vi "Migrate all Measurement Dependencies.vi"(0 "project path":path, 1 "measurement paths":path[](array[path]), 2 "init":T1[](array[typedef]), 5 "plug-in names":string[](array[string]), 7 "measurement dependencies":path[][](array[path]), 9 "outside items":string[](array[string]), 11 "error in":errorcluster, 12 "shared dependent vis":path[](array[path])) -> (6 "destination directory":path[](array[path]), 15 "error out":errorcluster)   [LabVIEW 2021, in "Multiple Converter.lvlib"]
uses:
  Multiple Converter.lvlib
  TypeDefs/Library Info.ctl
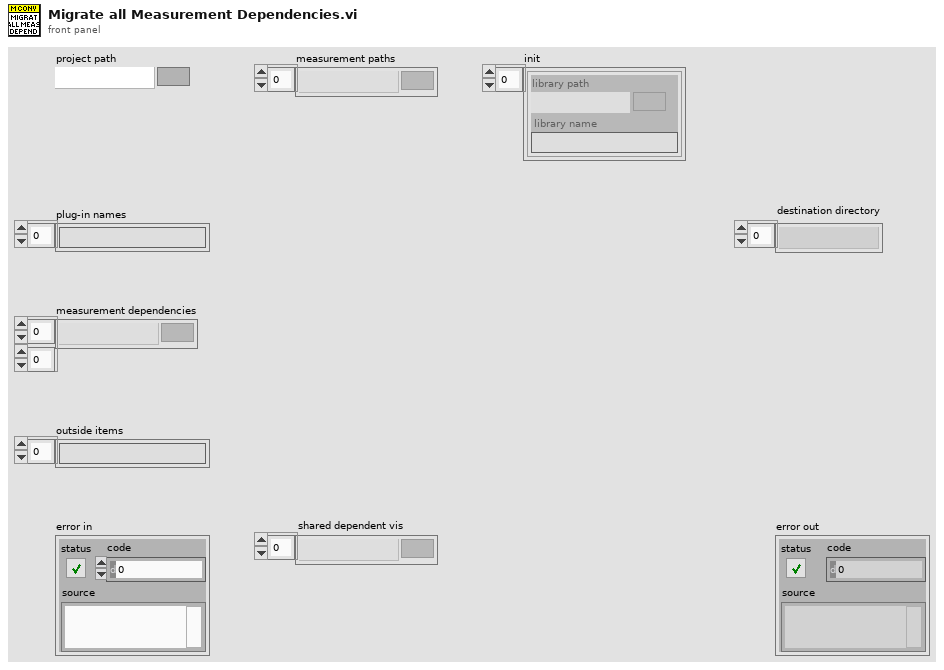
[diagram p1: front panel]
types:
  T1 = typedef "Multiple Converter.lvlib/Library Info.ctl" = cluster{"library path":path, "library name":string}
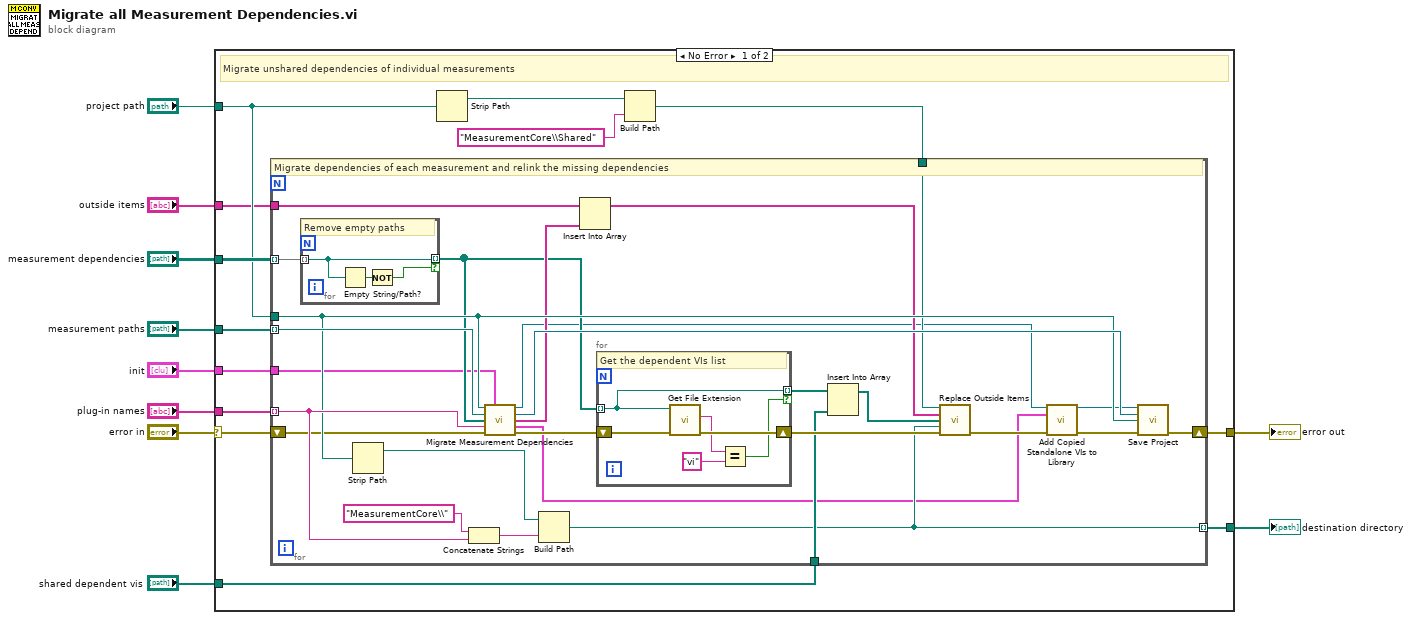
[diagram p0: block diagram]
diagram:
  n1 = case shown="No Error" "error in" {
    selector: "error in" -> [w22 w60]
    tunnel: "measurement dependencies" -> [w23 _]
    tunnel: "project path" -> [w18 _]
    tunnel: "outside items" -> [w17 _]
    tunnel: "measurement paths" -> [w16 _]
    tunnel: "plug-in names" -> [w15 _]
    tunnel: [w14 w60] -> w4
    tunnel: "shared dependent vis" -> [w13 _]
    tunnel: [w12 _] -> w2
    tunnel: "init" -> [w11 _]
    frame No Error {
      # "Migrate unshared dependencies of individual measurements"
      n2 = Strip Path(path=w18) -> (stripped path=w19:path)  [unwired: 1 out]
      n3 = Build Path(base path=w19, name or relative path="MeasurementCore\\Shared" ("string")) -> (appended path=w21:path)
      n4 = for {
        tunnel: w18 -> [w42]
        tunnel: w16 -> [w47] mode=indexing
        tunnel: w15 -> [w44] mode=indexing
        tunnel: w17 -> [w41]
        tunnel: w21 -> [w38]
        shift-right: [w48] -> w14
        shift-left: w22 -> [w37]
        tunnel: w23 -> [w36] mode=indexing
        tunnel: w13 -> [w31]
        tunnel: [w29] -> w12 mode=indexing
        tunnel: w11 -> [w28]
        # "Migrate dependencies of each measurement and relink the missing dependencies"
        n5 = for {
          tunnel: w36 -> [w58] mode=indexing
          tunnel: [w58] -> w33 mode=indexing if=w57
          # "Remove empty paths"
          n6 = Empty String/Path?(string/path=w58) -> (empty?=w59:bool)
          n7 = Not(x=w59) -> (.not. x?=w57:bool)
        }
        n8 = Strip Path(path=w42) -> (stripped path=w43:path)  [unwired: 1 out]
        n9 = Concatenate Strings("MeasurementCore\\" ("string"), w44) -> (w34:string)
        n10 = call "Migrate Measurement Dependencies.vi"("project path"=w42, "init"=w28, "measurement path"=w47, "dependencies path"=w33, "plug-in name"=w44, "error in"=w37) -> ("project reference"=w25:refnum<vi>, "measurement core reference"=w46:refnum<vi>, "outside items"=w40:string[], "copied standalone VIs"=w26:cluster{"Lib path":path, "VI path":path}[], "error out"=w50:errorcluster)  [unwired: 5 in]
        n11 = Build Path(base path=w43, name or relative path=w34) -> (appended path=w29:path)
        n12 = Insert Into Array(array=w41, new element=w40) -> (w39:string[])  [unwired: 1 in]
        n13 = for {
          shift-right: [w55] -> w35
          shift-left: w50 -> [w56]
          tunnel: w33 -> [w54] mode=indexing
          tunnel: [w54] -> w32 mode=indexing if=w51
          # "Get the dependent VIs list"
          n14 = call <vilib>:"Get File Extension.vi"("error in (no error)"=w56, "file"=w54) -> ("error out"=w55:errorcluster, "lowercase file extension"=w52:string)  [unwired: 5 in, 3 out]
          n15 = Equal?(x=w52, y="vi" ("x")) -> (x = y?=w51:bool)
        }
        n16 = Insert Into Array(array=w32, new element=w31) -> (w30:path[])  [unwired: 1 in]
        n17 = call "Replace Outside Items.vi"("shared directory"=w38, "outside vis"=w39, "dependent vis"=w30, "measurement directory"=w29, "error in"=w35) -> ("error out"=w49:errorcluster)  [unwired: 10 in]
        n18 = call "Add Copied Standalone VIs to Library.vi"("project reference in"=w25, "copied standalone VIs"=w26, "error in"=w49) -> ("project reference out"=w24:refnum<vi>, "error out"=w27:errorcluster)  [unwired: 11 in]
        n19 = call "Save Project.vi"("project reference"=w24, "measurement core reference"=w46, "project path"=w42, "error in"=w27) -> ("error out"=w48:errorcluster)  [unwired: 11 in]
      }
    }
    frame Error {
      # "Pass"
    }
  }
  "error out" <- w4
  "destination directory" <- w2
